vi "Open.vi"(8 "error in (no error)":errorcluster, 11 "User Connections in":refnum<class "User Connections.lvclass">) -> (0 "error out":errorcluster, 3 "User Connections out":refnum<class "User Connections.lvclass">)   [LabVIEW 2021, in "File Library.lvlib" / "User Connections.lvclass"]
uses:
  User Connections.lvclass
  User Connections.lvclass/User Connections.ctl
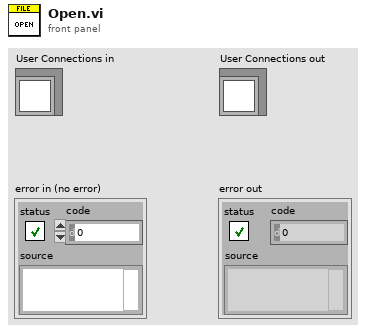
[diagram p1: front panel]
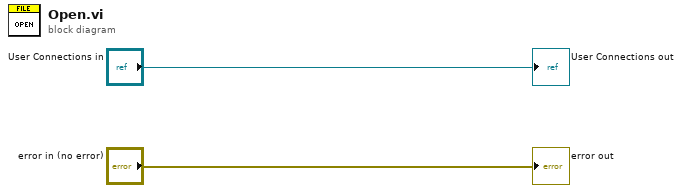
[diagram p0: block diagram]
diagram:
  "error out" <- "error in (no error)"
  "User Connections out" <- "User Connections in"
